vi "TestVI.vi"() -> ()   [LabVIEW 2021]
uses:
  Data_Cluster.ctl
  Measurement_Cluster.ctl
  Mode_Enum.ctl
panel:
  out "Mag B":dbl
  out "Temp T":dbl
  out "Waveform Graph 4":dbl[](graph)
  out "Waveform Graph 3":dbl[](graph)
  out "Waveform Graph 2":dbl[](graph)
  out "Time Stamp":timestamp
  out "data out":string
  out "Waveform Graph":dbl[](graph)
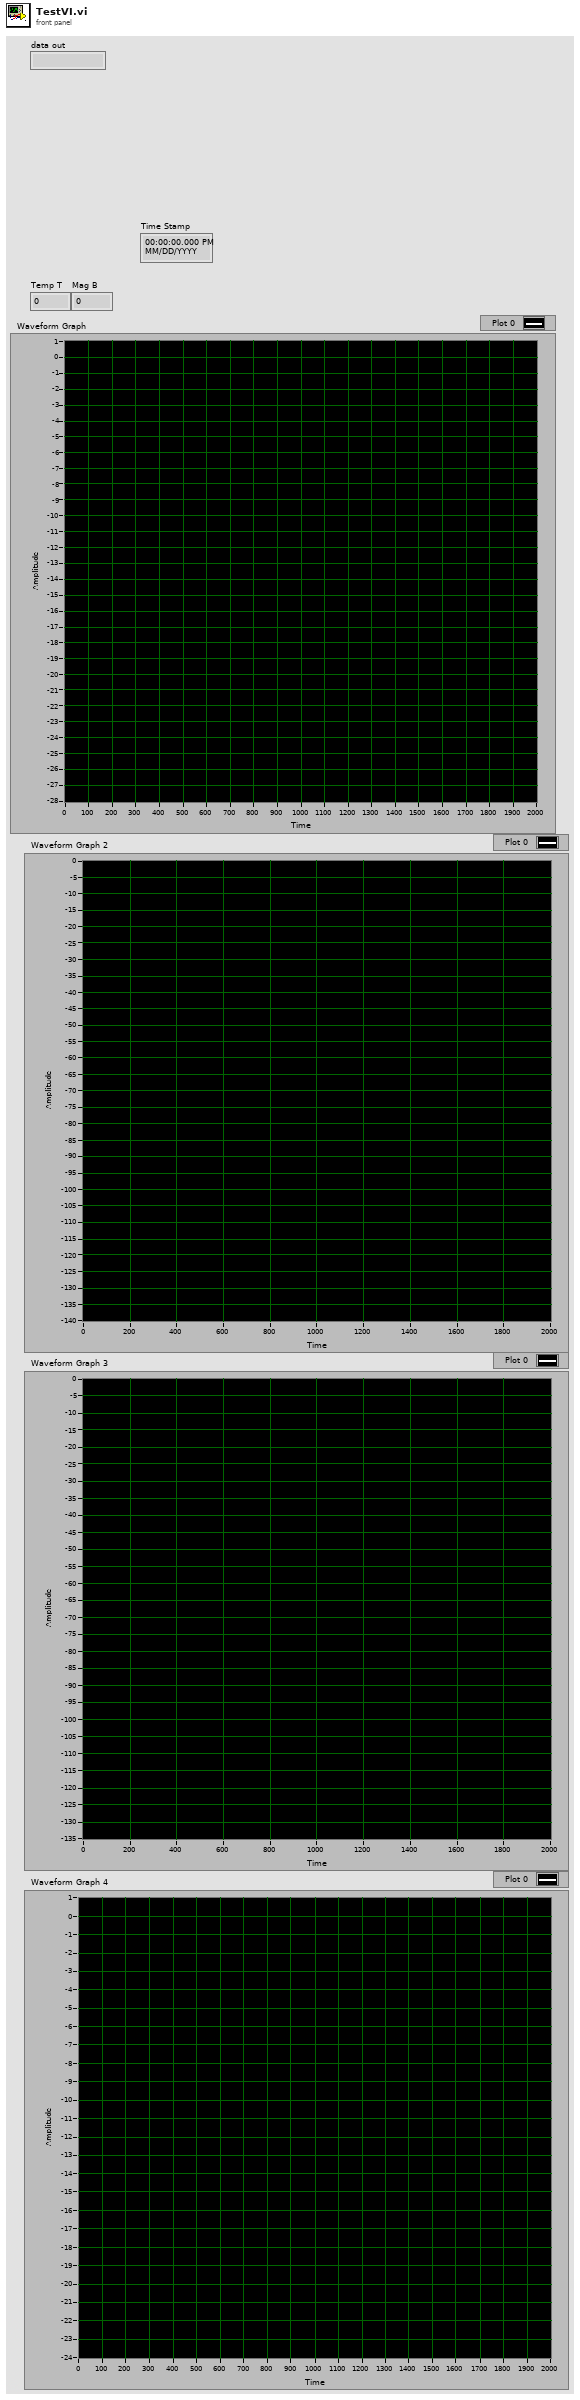
[diagram p1: front panel]
types:
  T1 = typedef "Data_Cluster.ctl" = cluster{"Value":dbl, "GUI Data Cluster":cluster{"S11":bool, "S21":bool, "S12":bool, "S22":bool, "S11Meas":enum16{"Log-magnitude (dB)", "Linear magnitude", "Phase (deg)", "Time Domain", "Real", "Imaginary", "Group Delay", "Polarlinear"}, "S21Meas":enum16{"Log-magnitude (dB)", "Linear magnitude", "Phase (deg)", "Time Domain", "Real", "Imaginary", "Group Delay", "Polarlinear"}, "S12Meas":enum16{"Log-magnitude (dB)", "Linear magnitude", "Phase (deg)", "Time Domain", "Real", "Imaginary", "Group Delay", "Polarlinear"}, "S22Meas":enum16{"Log-magnitude (dB)", "Linear magnitude", "Phase (deg)", "Time Domain", "Real", "Imaginary", "Group Delay", "Polarlinear"}}, "Timing":cluster{"Last Operation":dbl, "Stop @ T":bool, "Delta T Log":bool, "End T":dbl, "Delta T":dbl, "Last Temp":dbl}, "Measurements":T2[], "Hardware":cluster{"VNA TCP Con":refnum<k5>, "VNA TCP Port":i32, "Global T VAR":refnum<k21>, "Global B VAR":refnum<k21>}, "Operation":cluster{"Operation Mode":T3, "Status":string, "NewLog?":bool}}
  T2 = typedef "Measurement_Cluster.ctl" = cluster{"Time Stamp":timestamp, "Temp T":dbl, "Mag B":dbl, "VNA S11":dbl[], "VNA S21":dbl[], "VNA S12":dbl[], "VNA S22":dbl[]}
  T3 = typedef "Mode_Enum.ctl" = enum16{"OvenNRDY", "Logging", "Idle-Off", "Idle"}
  T4 = enum16{"Standard", "Buffered", "CRLF", "Immediate"}
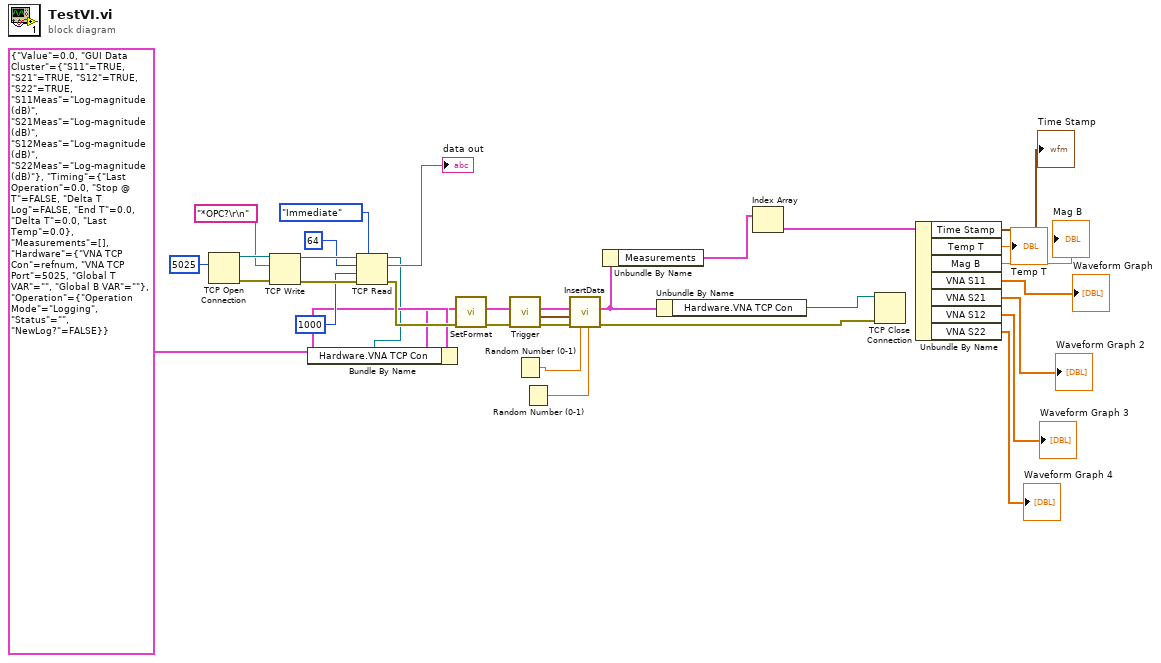
[diagram p0: block diagram]
diagram:
  n1 = TCP Open Connection(remote port or service name=u16 5025) -> (connection ID=w32:refnum<k5>, error out=w31:errorcluster)  [unwired: 4 in]
  n2 = TCP Write(connection ID=w32, data in="*OPC?\r\n", error in (no error)=w31) -> (connection ID out=w29:refnum<k5>, error out=w28:errorcluster)  [unwired: 1 in, 1 out]
  n3 = TCP Read(connection ID=w29, bytes to read=64, error in (no error)=w28, 7:T4."Immediate" ("mode (standard)"), 9:1000 ("timeout ms (25000)")) -> (connection ID out=w18:refnum<k5>, data out=→"data out":string, error out=w21:errorcluster)
  n4 = Bundle By Name(cluster=T1 {"Value"=0.0, "GUI Data Cluster"={"S11"=TRUE, "S21"=TRUE, "S12"=TRUE, "S22"=TRUE, "S11Meas"=enum."Log-magnitude (dB)", "S21Meas"=enum."Log-magnitude (dB)", "S12Meas"=enum."Log-magnitude (dB)", "S22Meas"=enum."Log-magnitude (dB)"}, "Timing"={"Last Operation"=0.0, "Stop @ T"=FALSE, "Delta T Log"=FALSE, "End T"=0.0, "Delta T"=0.0, "Last Temp"=0.0}, "Measurements"=[], "Hardware"={"VNA TCP Con"=refnum, "VNA TCP Port"=5025, "Global T VAR"="", "Global B VAR"=""}, "Operation"={"Operation Mode"=enum."Logging", "Status"="", "NewLog?"=FALSE}} ("VNACluster In"), "Hardware.VNA TCP Con"=w18) -> (w19:T1)
  n5 = call "SetFormat.vi"("error in (no error)"=w21, "VNACluster In"=w19) -> ("error out"=w22:errorcluster, "VNACluster Out"=w23:T1)  [unwired: 7 in, 1 out]
  n6 = call "Trigger.vi"("error in (no error)"=w22, "VNACluster In"=w23) -> ("error out"=w16:errorcluster, "TriggerTime"=w15:timestamp, "VNACluster Out"=w17:T1)  [unwired: 7 in]
  n7 = Random Number (0-1)() -> (number: 0 to 1=w2:dbl)
  n8 = Random Number (0-1)() -> (number: 0 to 1=w1:dbl)
  n9 = call "InsertData.vi"("Mag B"=w1, "Temp T"=w2, "Time Stamp"=w15, "error in (no error)"=w16, "VNACluster In"=w17) -> ("error out"=w13:errorcluster, "VNACluster Out"=w12:T1)  [unwired: 5 in]
  n10 = Unbundle By Name(w12) -> ("Measurements"=w11:T2[])
  n11 = Unbundle By Name(w12) -> ("Hardware.VNA TCP Con"=w14:refnum<k5>)
  n12 = Index Array(array=w11) -> (element=w10:T2)  [unwired: 1 in]
  n13 = TCP Close Connection(connection ID=w14, error in (no error)=w13) -> ()  [unwired: 1 in, 2 out]
  n14 = Unbundle By Name(w10) -> ("Time Stamp"=→"Time Stamp":timestamp, "Temp T"=→"Temp T":dbl, "Mag B"=→"Mag B":dbl, "VNA S11"=→"Waveform Graph":dbl[], "VNA S21"=→"Waveform Graph 2":dbl[], "VNA S12"=→"Waveform Graph 3":dbl[], "VNA S22"=→"Waveform Graph 4":dbl[])
